vi "剖面多参数组合(子VI).vi"(7 "数据值":string[](array[string])=["17.991", "52.06", "45.09", "0.02", "0.03"], 9 "层数":string="1", 10 "数据标识":string="N", 11 "数据类型":string="N") -> (3 "编码输出":string)   [LabVIEW 2016, in "数据传输系统.lvlib"]
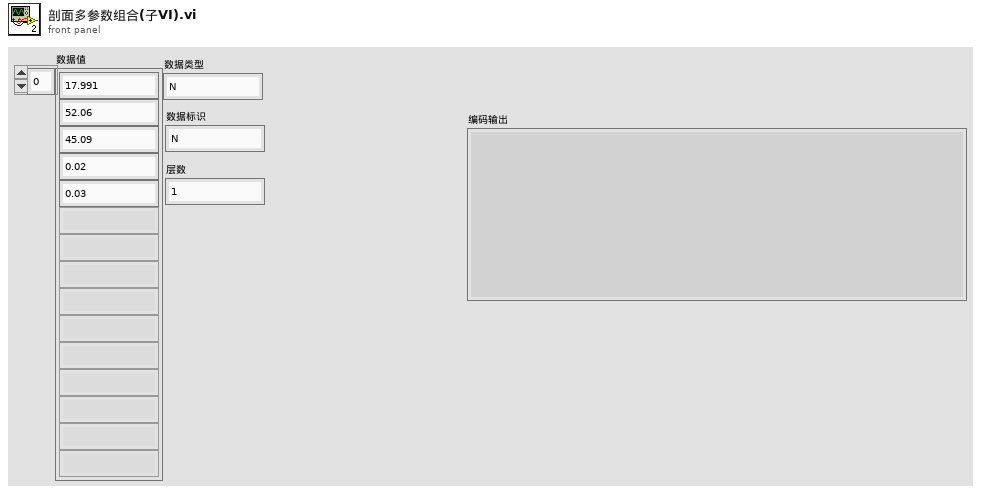
[diagram p1: front panel]
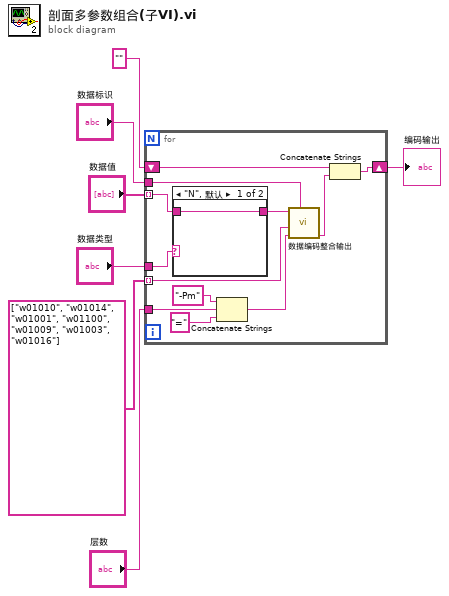
[diagram p0: block diagram]
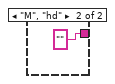
[diagram p2: hidden frame]
diagram:
  n1 = for {
    tunnel: "数据类型" -> [w15]
    tunnel: "层数" -> [w14]
    tunnel: "数据标识" -> [w13]
    tunnel: "数据值" -> [w12] mode=indexing
    shift-right: [w9] -> w4
    shift-left: "" ("编码输出") -> [w10]
    tunnel: string[] ["w01010", "w01014", "w01001", "w01100", "w01009", "w01003", "w01016"] -> [w8] mode=indexing
    n2 = case shown="\"N\", 默认" w15 {
      tunnel: [w20 ""] -> w18
      tunnel: w12 -> [w20 _]
      frame "N", Default {
      }
      frame "M", "hd" {
      }
    }
    n3 = Concatenate Strings("-Pm", w14, "=" ("字符串")) -> (w16:string)
    n4 = call "数据编码整合输出.vi"("数据标识"=w13, "数据类型"=w16, "污染物编码"=w8, "数据值"=w18) -> ("编码输出"=w11:string)  [unwired: 7 in]
    n5 = Concatenate Strings(w10, w11) -> (w9:string)
  }
  "编码输出" <- w4
